vi "Update Data Core.vi"(8 "error in":errorcluster, 11 "BNT_ULx-MCSV in":refnum<class "BNT_ULx-MCSV.lvclass">) -> (0 "error out":errorcluster, 2 "CSPP_DataCollection":refnum<class "CSPP_DataCollection.lvclass">, 3 "BNT_ULx-MCSV out":refnum<class "BNT_ULx-MCSV.lvclass">)   [LabVIEW 2020, in "BNT_ULx.lvlib" / "BNT_ULx-MCSV.lvclass"]
doc: "Read data and send to caller actor."
uses:
  BNT_ULx-MCSV.lvclass
  CSPP_Core/Classes/CSPP_BaseClasses/DataCollection/CSPP_DataCollection.lvclass
  BNT_ULx-MCSV.lvclass/BNT_ULx-MCSV.ctl
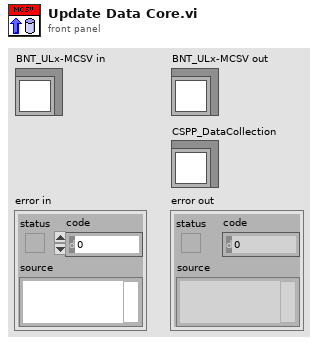
[diagram p1: front panel]
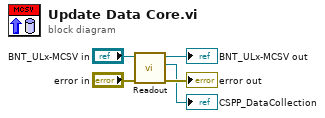
[diagram p0: block diagram]
diagram:
  n1 = call "Readout.vi"("Error In"="error in", "BNT_ULx-MCSV in"="BNT_ULx-MCSV in") -> ("Error Out"=→"error out":errorcluster, "CSPP_DataCollection out"=→"CSPP_DataCollection":refnum<class "CSPP_DataCollection.lvclass">, "BNT_ULx-MCSV out"=→"BNT_ULx-MCSV out":refnum<class "BNT_ULx-MCSV.lvclass">)  [unwired: 7 in]
